vi "aft_ANC_Dotproduct (FXP).vi"(5 "enable(F)":bool, 7 "reset(F)":bool, 11 "data in":fxp<+/-,64,4>) -> (3 "data out":fxp<+/-,32,4> format="%.30g")   [LabVIEW 2023]
doc: "This VI is an integrator.\n\nThis VI is an instance VI. Complete the following steps to convert this instance VI into a subVI.\n\n(1) Right-click the instance VI.\n(2) Select <b>Open Front Panel</b> from the shortcut menu.\n(3) Save the VI."
uses:
  <vilib>/rvi/FXPMathLib/FxpConvert/subVIs/nifxpmath_Convert_SimConfig.ctl
  <vilib>/fxp/LVFixedPointQuantizationPolicyTypeDef.ctl
  <vilib>/fxp/LVFixedPointOverflowPolicyTypeDef.ctl
  <vilib>/rvi/FXPMathLib/FxpConvert/simVIs/DllFxpConvertTemp_sub.vi
  <vilib>/rvi/FXPMathLib/FxpAdd/XNode/nifxpmath_Add.xnode
  <vilib>/rvi/FXPMathLib/FxpConvert/XNode/nifxpmath_Convert.xnode
  <vilib>/rvi/FXPMathLib/sim/FxpSim.dll
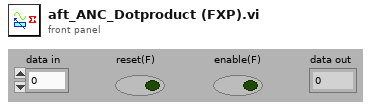
[diagram p1: front panel]
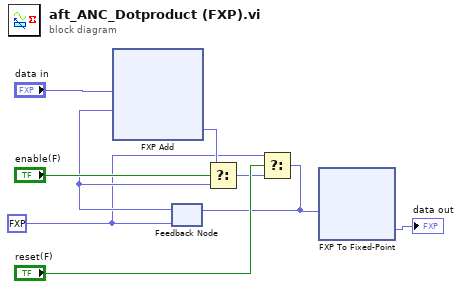
[diagram p0: block diagram]
diagram:
  w1 = fxp<+/-,64,4> 0.0 ("data in 2")
  n1 = feedback #1(w1) -> (w5:fxp<+/-,64,4>)
  n2 = xnode "FXP Add"("x"="data in", "y"=w5) -> ("x+y"=w6:fxp<+/-,64,4>)
  n3 = Select(t=w6, s="enable(F)", f=w5) -> (s? t:f=w4:fxp<+/-,64,4>)
  n4 = Select(t=w1, s="reset(F)", f=w4) -> (s? t:f=w3:fxp<+/-,64,4>)
  n5 = feedback-in #1(w3) -> ()
  n6 = xnode "FXP To Fixed-Point"("x"=w3) -> ("y"=→"data out":fxp<+/-,32,4>)
